vi "transHexaPosCoorSys.vi"(8 "error in (no error)":errorcluster, 10 "Hex Pos":dbl[](array[numeric]), 11 "SubSysAdap in":refnum<class "SubSysAdap.lvclass">) -> (0 "error out":errorcluster, 2 "Trans Hex Pos":dbl[](array[numeric]), 3 "SubSysAdap out":refnum<class "SubSysAdap.lvclass">)   [LabVIEW 2016, in "OfcFunc.lvlib" / "SubSysAdap.lvclass"]
doc: "Transform the hexapod position between the Zemax and subsystem coordinate system. Zemax coordinate is (z', x', y', rx', ry') and the hexapod is (x, y, z, rx, ry, rz)."
uses:
  SubSysAdap.lvclass
  SubSysAdap.lvclass/SubSysAdap.ctl
  <vilib>/Analysis/_algsub.llb/Real PseudoInverse Matrix.vi
  <vilib>/Analysis/Matrix/Numeric/Conversions/Array To Matrix - RA2.vi
  <vilib>/Analysis/Matrix/Numeric/Conversions/Matrix To Array - RM.vi
  <vilib>/Analysis/NI_AALPro.lvlib
  <vilib>/Analysis/Matrix/NI_Matrix.lvlib
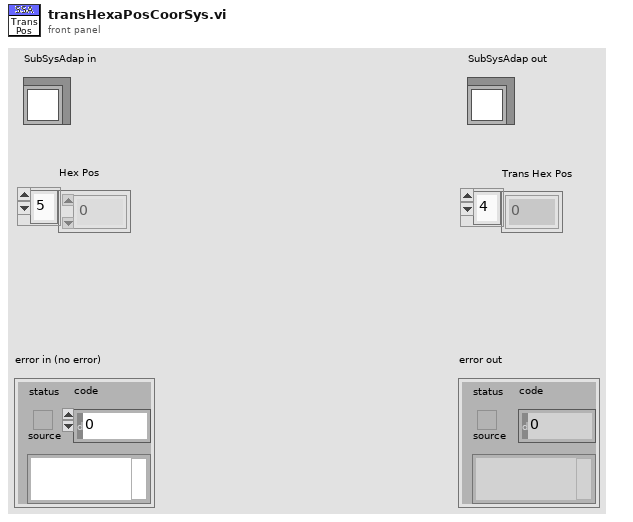
[diagram p1: front panel]
types:
  T1 = typedef "NI_Matrix.lvlib/RealMatrix.ctl" = dbl[][]
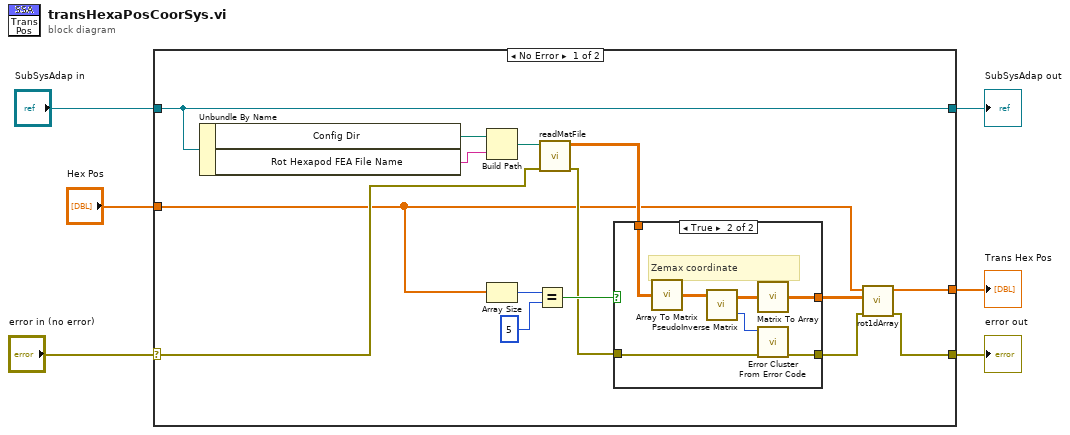
[diagram p0: block diagram]
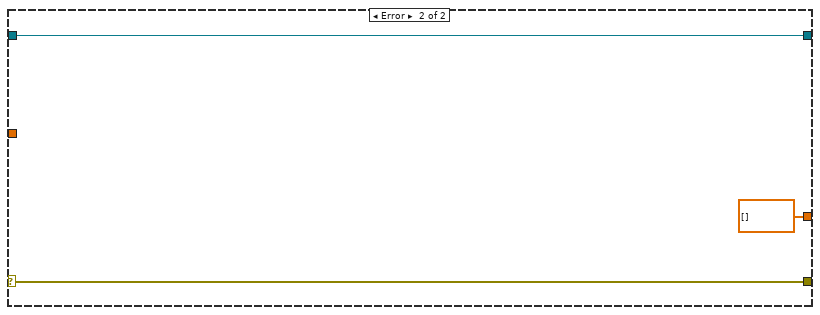
[diagram p3: hidden frame]
diagram:
  n1 = case shown="No Error" "error in (no error)" {
    selector: "error in (no error)" -> [w12 w33]
    tunnel: [w8 w33] -> w5
    tunnel: [w21 w32] -> w3
    tunnel: "SubSysAdap in" -> [w21 w32]
    tunnel: "Hex Pos" -> [w10 _]
    tunnel: [w7 dbl[] [] ("Rotated 1D Array")] -> w1
    frame No Error {
      n2 = Unbundle By Name(w21) -> ("Config Dir"=w20:path, "Rot Hexapod FEA File Name"=w19:string)
      n3 = Build Path(base path=w20, name or relative path=w19) -> (appended path=w18:path)
      n4 = Array Size(array=w10) -> (size(s)=w17:i32)
      n5 = Equal?(x=w17, y=5) -> (x = y?=w15:bool)
      n6 = call "readMatFile.vi"("error in (no error)"=w12, "Path"=w18) -> ("error out"=w11:errorcluster, "Matrix"=w14:dbl[][])  [unwired: 8 in]
      n7 = case shown="True" w15 {
        tunnel: w14 -> [w23 w30]
        tunnel: [w23 w27] -> w13
        tunnel: w11 -> [w22 w25]
        tunnel: [w22 w24] -> w9
        frame False {
          # "Optical coordinate"
        }
        frame True {
          # "Zemax coordinate"
          n8 = call-poly <vilib>:"Array To Matrix.vi"("Real 2D Array"=w30) -> ("Real Matrix"=w29:T1)
          n9 = call-poly <vilib>:"PseudoInverse Matrix.vi"("Input Matrix"=w29) -> ("error"=w26:i32, "PseudoInverse Matrix"=w28:T1)  [unwired: 1 in]
          n10 = call-poly <vilib>:"Matrix To Array.vi"("Real Matrix"=w28) -> ("Real 2D Array"=w27:dbl[][])
          n11 = call <vilib>:"Error Cluster From Error Code.vi"("error in (no error)"=w25, "error code (0)"=w26) -> ("error out"=w24:errorcluster)  [unwired: 7 in]
        }
      }
      n12 = call "rot1dArray.vi"("error in (no error)"=w9, "Rot Mat"=w13, "1D Array"=w10) -> ("error out"=w8:errorcluster, "Rotated 1D Array"=w7:dbl[])  [unwired: 7 in]
    }
    frame Error {
    }
  }
  "error out" <- w5
  "SubSysAdap out" <- w3
  "Trans Hex Pos" <- w1
